vi "compass_EWSN.vi"(4 "center":cluster{"x":i32, "y":i32}={"x"=40, "y"=40}, 6 "size":i16=30, 8 "angle":dbl(slide)=-67.31238145757612 scale=-180.0..180.0, 10 "pict in":picture) -> (3 "pict out":picture)   [LabVIEW 2017]
uses:
  <vilib>/Analysis/baseanly.llb/Real A x B.vi
  <vilib>/Analysis/baseanly.llb/A x Vector.vi
  <vilib>/Analysis/NI_AALBase.lvlib
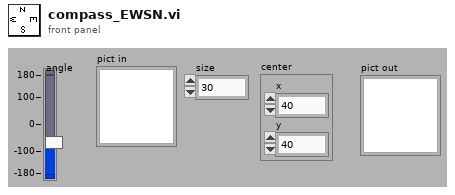
[diagram p1: front panel]
types:
  T1 = typedef "NI_Matrix.lvlib/RealMatrix.ctl" = dbl[][]
  T2 = cluster{"A x Vector[0]":dbl, "A x Vector[1]":dbl}
  T3 = cluster{"A x Vector[0]":dbl, "A x Vector[1]":dbl}[]
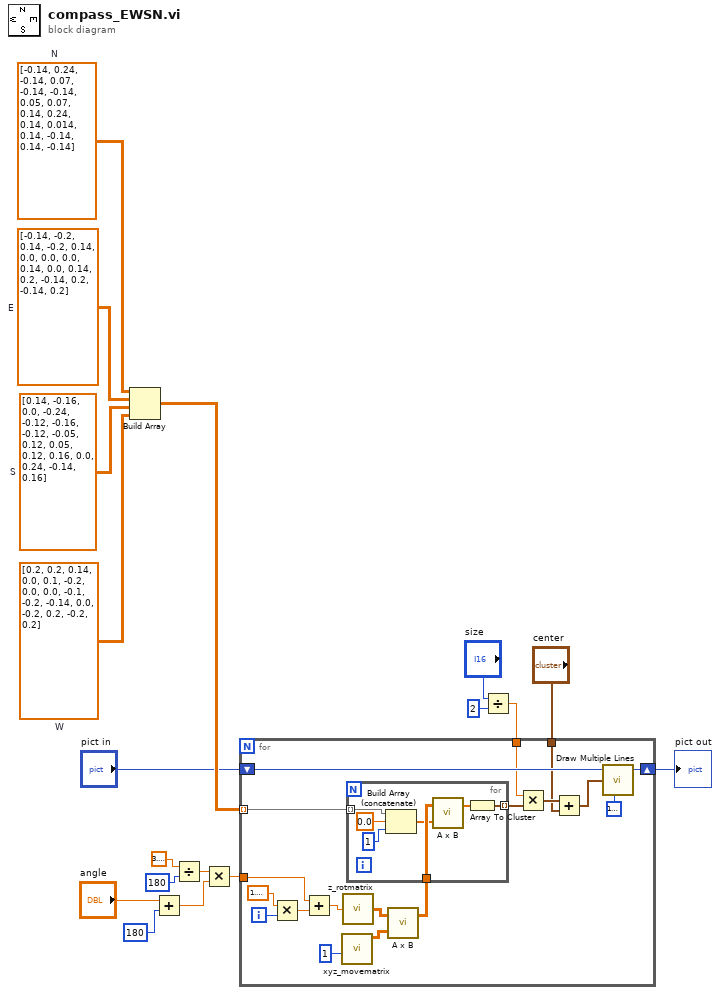
[diagram p0: block diagram]
diagram:
  w9 = dbl[][] [[0.14, -0.16], [0.0, -0.24], [-0.12, -0.16], [-0.12, -0.05], [0.12, 0.05], [0.12, 0.16], [0.0, 0.24], [-0.14, 0.16]]  # S
  w10 = dbl[][] [[0.2, 0.2], [0.14, 0.0], [0.1, -0.2], [0.0, 0.0], [-0.1, -0.2], [-0.14, 0.0], [-0.2, 0.2], [-0.2, 0.2]]  # W
  w6 = dbl[][] [[-0.14, -0.2], [0.14, -0.2], [0.14, 0.0], [0.0, 0.0], [0.14, 0.0], [0.14, 0.2], [-0.14, 0.2], [-0.14, 0.2]]  # E
  w7 = dbl[][] [[-0.14, 0.24], [-0.14, 0.07], [-0.14, -0.14], [0.05, 0.07], [0.14, 0.24], [0.14, 0.014], [0.14, -0.14], [0.14, -0.14]]  # N
  n1 = Build Array(w7, w6, w9, w10) -> (w8:dbl[][][])
  n2 = Add(x="angle", y=180) -> (x+y=w2:dbl)
  n3 = Divide(x=3.141592653589793, y=180) -> (x/y=w15:dbl)
  n4 = Multiply(x=w15, y=w2) -> (x*y=w12:dbl)
  n5 = Divide(x="size", y=2 ("y 2")) -> (x/y=w18:dbl)
  n6 = for {
    tunnel: w8 -> [w35] mode=indexing
    shift-right: [w29] -> w4
    shift-left: "pict in" -> [w28]
    tunnel: "center" -> [w24]
    tunnel: w12 -> [w23]
    tunnel: w18 -> [w21]
    i -> [w27]
    n7 = Multiply(x=1.5707963267948966, y=w27) -> (x*y=w19:dbl)
    n8 = Add(x=w23, y=w19) -> (x+y=w25:dbl)
    n9 = call "xyz_movematrix.vi"("y"=1) -> ("matrix out"=w31:dbl[][])  [unwired: 6 in]
    n10 = call "z_rotmatrix.vi"("z-angle"=w25) -> ("z-matrix"=w32:dbl[][])
    n11 = call-poly <vilib>:"A x B.vi"("B"=w31, "A"=w32) -> ("A x B"=w33:T1)  [unwired: 1 out]
    n12 = for {
      tunnel: w35 -> [w43] mode=indexing
      tunnel: [w40] -> w36 mode=indexing
      tunnel: w33 -> [w39]
      n13 = Build Array (concatenate)(w43, 0.0 ("Slide"), 1 ("Slide")) -> (w38:dbl[])
      n14 = call-poly <vilib>:"A x B.vi"("Vector"=w38, "A"=w39) -> ("A x Vector"=w37:dbl[])  [unwired: 1 out]
      n15 = Array To Cluster(array=w37) -> (cluster=w40:T2)
    }
    n16 = Multiply(x=w21, y=w36) -> (x*y=w34:T3)
    n17 = Add(x=w34, y=w24) -> (x+y=w30:cluster{dbl, dbl}[])
    n18 = call <vilib>:"Draw Multiple Lines.vi"("picture"=w28, "line endpoints"=w30, "color(black)"=u32 16777226) -> ("new picture"=w29:picture)  [unwired: 6 in]
  }
  "pict out" <- w4
